vi "RecvFrom().vi"(8 "Error In":errorcluster, 11 "Socket To Use":u32 format="%08x") -> (0 "Error Out":errorcluster, 1 "RxTimeStamp":u32, 2 "Bytes Read":i32, 3 "Socket Out":u32 format="%08x", 4 "Sending IP":string, 5 "Received IP Packet":u8[](array[numeric]) format="%02x")   [LabVIEW 2018]
uses:
  ws2_32.dll
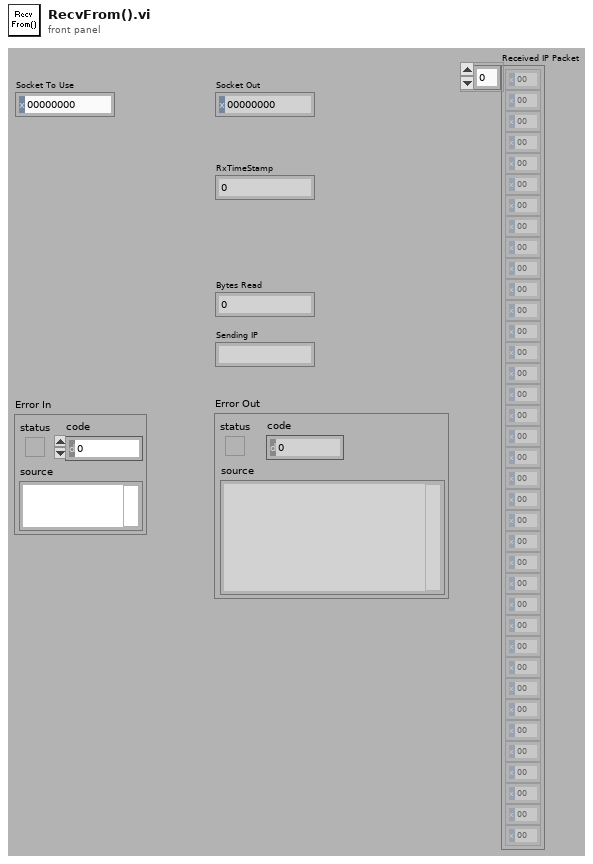
[diagram p1: front panel]
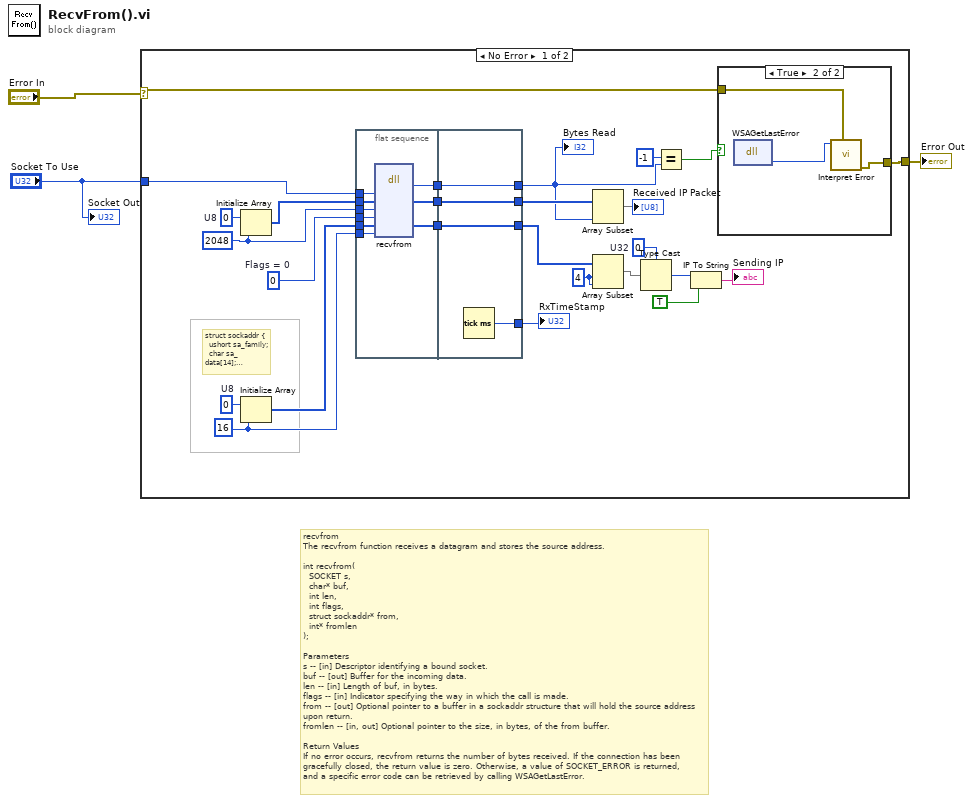
[diagram p0: block diagram]
diagram:
  # "recvfrom\nThe recvfrom function receives a datagram and stores the source address.\n\nint recvfrom(\n  SOCKET s,\n  char* buf,\n  int len,\n  int flags,\n  struct sockaddr* from,\n  int* fromlen\n);\n\nParameters\ns -- [in] Descriptor identifying a bound socket. \nbuf -- [out] Buffer for the incoming data. \nlen -- [in] Length of buf, in bytes. \nflags -- [in] Indicator specifying the way in which the call is made. \nfrom -- [out] Optional pointer to a buffer in a sockaddr structure that will hold the source address upon return. \nfromlen -- [in, out] Optional pointer to the size, in bytes, of the from buffer. \n\nReturn Values\nIf no error occurs, recvfrom returns the number of bytes received. If the connection has been \ngracefully closed, the return value is zero. Otherwise, a value of SOCKET_ERROR is returned, \nand a specific error code can be retrieved by calling WSAGetLastError."
  n1 = case shown="No Error" "Error In" {
    selector: "Error In" -> [w10 w47]
    tunnel: [w20 w47] -> w3
    tunnel: "Socket To Use" -> [w6 _]
    frame No Error {
      w22 = u8 0  # U8
      w25 = u8 0  # U8
      w15 = 4 ("index")
      w14 = u32 0  # U32
      w4 = 16 ("dimension size")
      w23 = 2048 ("dimension size")
      w26 = 0  # Flags = 0
      # "struct sockaddr {\n  ushort sa_family;\n  char sa_data[14];\n} ;"
      n2 = Initialize Array(w25, w23) -> (w24:u8[])
      n3 = Initialize Array(w22, w4) -> (w21:u8[])
      n4 = flat-sequence {
        tunnel: w4 -> [w32]
        tunnel: w21 -> [w33]
        tunnel: w23 -> [w34]
        tunnel: w24 -> [w35]
        tunnel: w26 -> [w36]
        tunnel: w6 -> [w38]
        tunnel: [w37] -> w9
        tunnel: [w31] -> w8
        tunnel: [w30] -> w7
        tunnel: [w39] -> w5
        tunnel: [w40] -> w11
        tunnel: [w41] -> w16
        tunnel: [w42] -> w27
        tunnel: w9 -> [w42]
        tunnel: w8 -> [w41]
        tunnel: w7 -> [w40]
        frame #0 {
          n5 = dll-call lib="ws2_32.dll" fn="recvfrom"("Socket to Use"=w38, "Receive Buffer"=w35, "Length of Buffer"=w34, "Flags"=w36, "From"=w33, "Fromlen"=w32) -> (w30:i32, "Receive Buffer"=w37:u8[], "From"=w31:u8[])  [unwired: 7 in, 2 out]
        }
        frame #1 {
          n6 = Tick Count (ms)() -> (millisecond timer value=w39:u32)
        }
      }
      n7 = Array Subset(array=w27, length=w11) -> (→"Received IP Packet":u8[])  [unwired: 1 in]
      n8 = Array Subset(array=w16, index=w15, length=w15) -> (w18:u8[])
      n9 = Type Cast(type=w14, x=w18) -> (*(type *) &x=w17:u32)
      n10 = Equal?(x=-1, y=w11) -> (x = y?=w28:bool)
      n11 = IP To String(1:TRUE ("dot notation? (F)"), 2:w17) -> (0:→"Sending IP":string)
      n12 = case shown="True" w28 {
        tunnel: w10 -> [w43 w45]
        tunnel: [w43 w44] -> w20
        frame False {
        }
        frame True {
          n13 = dll-call lib="ws2_32.dll" fn="WSAGetLastError"() -> (w46:i32)  [unwired: 3 in, 2 out]
          n14 = call "Interpret Error.vi"("Error In"=w45, "Code"=w46) -> ("Error Out"=w44:errorcluster)  [unwired: 9 in]
        }
      }
      "Bytes Read" <- w11
      "RxTimeStamp" <- w5
    }
    frame Error {
    }
  }
  "Error Out" <- w3
  "Socket Out" <- "Socket To Use"
